vi "Waveform to DVR.vi"(7 "gRPC Waveform Enabled":bool, 8 "error in (no error)":errorcluster, 10 "Waveform In":waveform(dbl)[](array[waveform]), 11 "gRPC Waveform Monitor in":T1) -> (0 "error out":errorcluster, 2 "Waveform Out":waveform(dbl)[](array[waveform]), 3 "gRPC Waveform Monitor out":T1)   [LabVIEW 2021, in "CIFWaveformMonitorWrapper.lvlib"]
uses:
  CIFWaveformMonitorWrapper.lvlib
  Typedef/WDT Array DVR.ctl
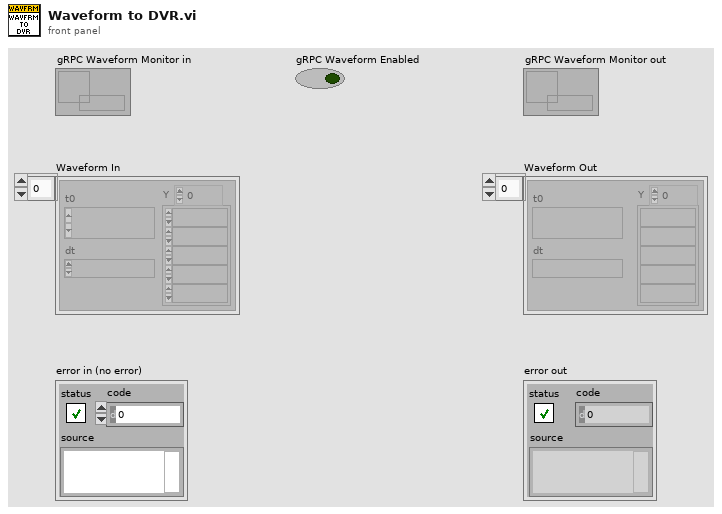
[diagram p1: front panel]
types:
  T1 = typedef "CIFWaveformMonitorWrapper.lvlib/WDT Array DVR.ctl" = refnum<data-value>
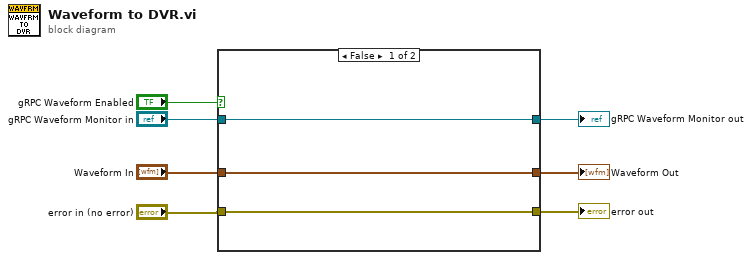
[diagram p0: block diagram]
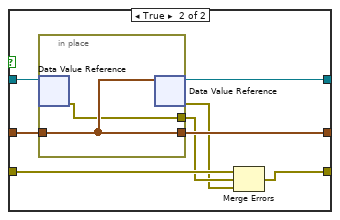
[diagram p2: hidden frame]
diagram:
  n1 = case shown="False" "gRPC Waveform Enabled" {
    tunnel: "gRPC Waveform Monitor in" -> [w8 w18]
    tunnel: "Waveform In" -> [w10 w17]
    tunnel: [w10 w16] -> w4
    tunnel: "error in (no error)" -> [w9 w15]
    tunnel: [w9 w12] -> w5
    tunnel: [w8 w11] -> w2
    frame False {
    }
    frame True {
      n2 = in-place {
        in-place-border: w17 -> [w20]
        in-place-border: [w20] -> w16
        in-place-border: [w19] -> w14
        n3 = in-place-dvr #1(w18) -> (w19:errorcluster)  [unwired: 1 out]
        n4 = in-place-dvr #1(w20) -> (w11:T1, w13:errorcluster)
      }
      n5 = Merge Errors(w15, w14, w13) -> (w12:errorcluster)
    }
  }
  "error out" <- w5
  "Waveform Out" <- w4
  "gRPC Waveform Monitor out" <- w2
